vi "niRFUtil MT UTIL Filter Taps - Gaussian Pulse.vi"(0 "Samples Per Symbol (16)":i32=16, 5 "Filter Length (3)":i32=3, 7 "Alpha (0.5)":dbl=0.5 format="%.2f", 11 "error in (no error)":errorcluster) -> (4 "Filter Coefficients":T1 min=0 max=127 format="%.2f", 15 "error out":errorcluster)   [LabVIEW 2015, in "niRFUtil.lvlib"]
doc: "This VI generates a Gaussian filter. \n\nB is the bandwidth in Hz\nT is the symbol period in symbols/sec\nOversampling Factor is the number of samples/symbol\nFilter Duration is the length of the filter in multiples of the symbol period. If odd, this number is coerced to the next largest even number."
uses:
  niRFUtil.lvlib
  Includes/niRFUtil INC Real Array.ctl
  <vilib>/Analysis/1siggen.llb/Ramp Pattern by Samples.vi
  <vilib>/Analysis/NI_AALBase.lvlib
panel:
  out "pulse":sgl[](graph)
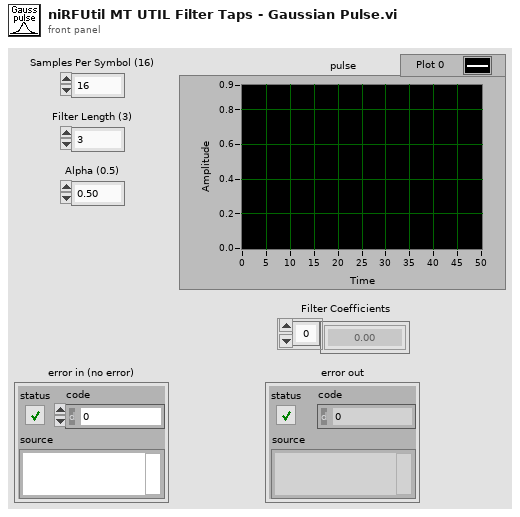
[diagram p1: front panel]
types:
  T1 = typedef "niRFUtil.lvlib/niRFUtil INC Real Array.ctl" = sgl[]
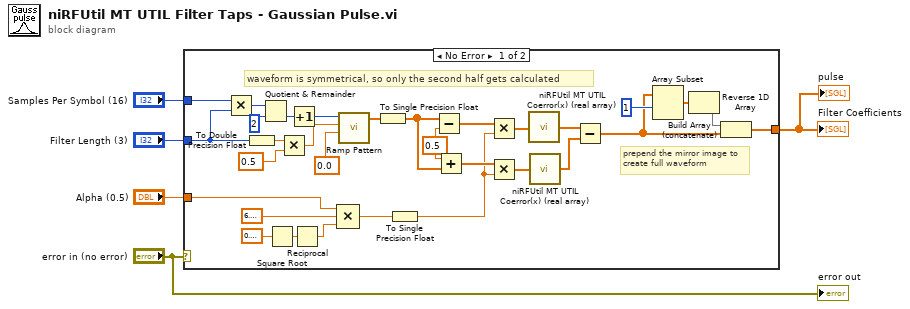
[diagram p0: block diagram]
diagram:
  n1 = case shown="No Error" "error in (no error)" {
    tunnel: "Alpha (0.5)" -> [w30 _]
    tunnel: "Samples Per Symbol (16)" -> [w10 _]
    tunnel: "Filter Length (3)" -> [w9 _]
    tunnel: [w8 _] -> w2
    frame No Error {
      w24 = sgl 0.5 ("start")
      # "prepend the mirror image to create full waveform"
      # "waveform is symmetrical, so only the second half gets calculated"
      n2 = Multiply(x=w10, y=w9) -> (x*y=w36:i32)
      n3 = To Double Precision Float(number=w9) -> (double precision float=w27:dbl)
      n4 = Quotient & Remainder(x=w36, y=2) -> (floor(x/y)=w34:i32)  [unwired: 1 out]
      n5 = Square Root(x=0.6931471805599453) -> (sqrt(x)=w31:dbl)
      n6 = Multiply(x=w27, y=sgl 0.5 ("start")) -> (x*y=w20:dbl)
      n7 = Increment(x=w34) -> (x+1=w28:i32)
      n8 = Reciprocal(x=w31) -> (1/x=w29:dbl)
      n9 = Compound Arithmetic op=MULTIPLY(w30, 6.283185307179586, w29) -> (w21:dbl)
      n10 = call-poly <vilib>:"Ramp Pattern.vi"("start"=sgl 0.0, "end"=w20, "samples"=w28) -> ("Ramp Pattern"=w25:dbl[])  [unwired: 7 in, 1 out]
      n11 = To Single Precision Float(number=w25) -> (single precision float=w7:sgl[])
      n12 = To Single Precision Float(number=w21) -> (single precision float=w6:sgl)
      n13 = Subtract(x=w7, y=w24) -> (x-y=w23:sgl[])
      n14 = Add(x=w24, y=w7) -> (x+y=w22:sgl[])
      n15 = Multiply(x=w23, y=w6) -> (x*y=w14:sgl[])
      n16 = Multiply(x=w22, y=w6) -> (x*y=w13:sgl[])
      n17 = call "niRFUtil MT UTIL Coerror(x) (real array).vi"("x"=w14) -> ("Coerror(x)"=w12:T1)
      n18 = call "niRFUtil MT UTIL Coerror(x) (real array).vi"("x"=w13) -> ("Coerror(x)"=w11:T1)
      n19 = Subtract(x=w12, y=w11) -> (x-y=w15:T1)
      n20 = Array Subset(array=w15, index=1 ("Array Index")) -> (w17:T1)  [unwired: 1 in]
      n21 = Reverse 1D Array(array=w17) -> (reversed array=w16:T1)
      n22 = Build Array (concatenate)(w16, w15) -> (w8:T1)
    }
    frame Error {
    }
  }
  "pulse" <- w2
  "Filter Coefficients" <- w2
  "error out" <- "error in (no error)"
